vi "DSF.Engine.Transfer.Set VS Channels Pointer.vi"(10 "VS Channels Pointer":refnum<class "DSF.Engine.Pointer.VS Channels.lvclass">, 11 "Transfer in":refnum<class "DSF.Engine.Transfer.lvclass">) -> (3 "Transfer out":refnum<class "DSF.Engine.Transfer.lvclass">)   [LabVIEW 2016, in "DSF.Engine.lvlib" / "DSF.Engine.Transfer.lvclass"]
uses:
  DSF.Engine.Transfer.lvclass
  Pointer/DSF.Engine.Pointer.VS Channels.lvclass
  DSF.Engine.Transfer.lvclass/DSF.Engine.Transfer.ctl
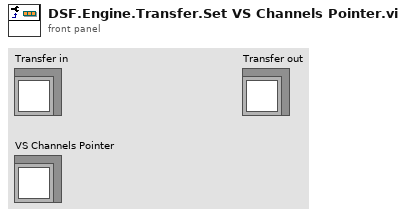
[diagram p1: front panel]
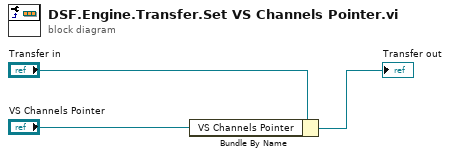
[diagram p0: block diagram]
diagram:
  n1 = Bundle By Name(cluster="Transfer in", "VS Channels Pointer"="VS Channels Pointer") -> (→"Transfer out":refnum<class "DSF.Engine.Transfer.lvclass">)
